vi "zadanie_1.vi"() -> ()   [LabVIEW 2017]
panel:
  out "Do 2":dbl
  out "Od 2":dbl
  out "XY Graph":cluster{"Y":dbl[], "Y":dbl[]}[](graph)
  in  "?":bool
  in  "Do":dbl
  in  "Od":dbl
  in  "b_2":dbl
  in  "a_2":dbl
  in  "b":dbl
  in  "a":dbl
  # "y1=ax+b"
  # "y2=ax+b"
  # "Przedzial argumentu x"
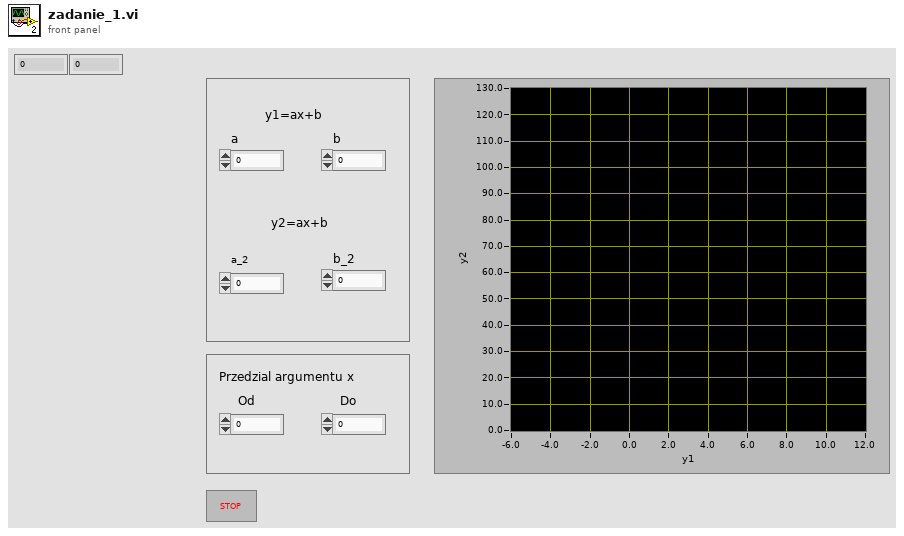
[diagram p1: front panel]
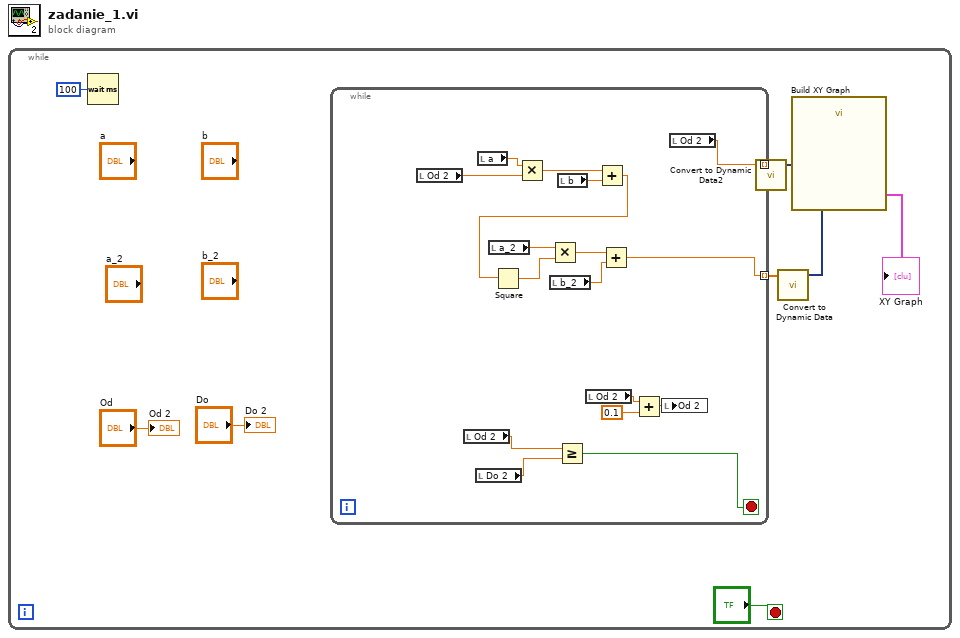
[diagram p0: block diagram]
diagram:
  n1 = while {
    stop <- "?" stop-if-true
    n2 = Wait (ms)(milliseconds to wait=u32 100) -> ()  [unwired: 1 out]
    n3 = while {
      tunnel: [w16] -> w7 mode=indexing
      tunnel: [w11] -> w5 mode=indexing
      stop <- w24 stop-if-true
      n4 = local read "Od 2"() -> (w14:dbl)
      n5 = local read "Od 2"() -> (w26:dbl)
      n6 = local read "Do 2"() -> (w25:dbl)
      n7 = local read "a"() -> (w15:dbl)
      n8 = local read "a_2"() -> (w19:dbl)
      n9 = Multiply(x=w15, y=w14) -> (x*y=w13:dbl)
      n10 = local read "b_2"() -> (w17:dbl)
      n11 = Greater Or Equal?(x=w26, y=w25) -> (x >= y?=w24:bool)
      n12 = local read "b"() -> (w12:dbl)
      n13 = local read "Od 2"() -> (w23:dbl)
      n14 = Add(x=w13, y=w12) -> (x+y=w10:dbl)
      n15 = Square(x=w10) -> (x^2=w20:dbl)
      n16 = Multiply(x=w19, y=w20) -> (x*y=w18:dbl)
      n17 = Add(x=w18, y=w17) -> (x+y=w16:dbl)
      n18 = Add(x=w23, y=0.1) -> (x+y=w21:dbl)
      n19 = local write "Od 2"(w21) -> ()
      n20 = local read "Od 2"() -> (w11:dbl)
    }
    n21 = call "Convert to Dynamic Data2"("Array"=w5) -> ("Dynamic Data Type"=w4:dynamicdata)  [unwired: 3 in]
    n22 = call "Convert to Dynamic Data"("Array"=w7) -> ("Dynamic Data Type"=w6:dynamicdata)  [unwired: 3 in]
    n23 = call "Build XY Graph"("Y Input"=w6, "X Input"=w4) -> ("XY Graph"=→"XY Graph":cluster{"X":dbl[], "Y":dbl[]}[])  [unwired: 8 in, 1 out]
    "Od 2" <- "Od"
    "Do 2" <- "Do"
  }
